vi "Wait on State.vi"(8 "error in (no error)":errorcluster, 9 "Timeout ms (-1)":i32=-1, 10 "Connection State":T1, 11 "VISA Client in":refnum<class "Serial Client.lvclass">) -> (0 "error out":errorcluster, 1 "Timed Out?":bool, 3 "VISA Client out":refnum<class "Serial Client.lvclass">)   [LabVIEW 2020, in "Stream-Serial.lvlib" / "Serial Client.lvclass"]
uses:
  Serial Client.lvclass
  Connection State.ctl
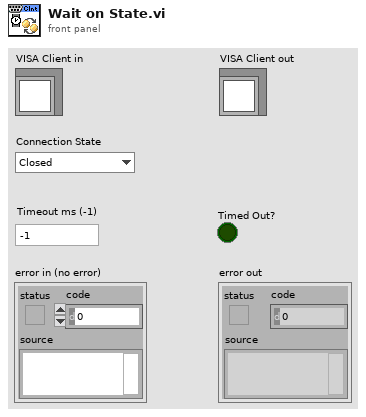
[diagram p1: front panel]
types:
  T1 = typedef "Stream-Serial.lvlib/Serial Client.lvclass/Connection State.ctl" = enum16{"Closed", "Idle", "Connecting", "Connected", "Shutdown"}
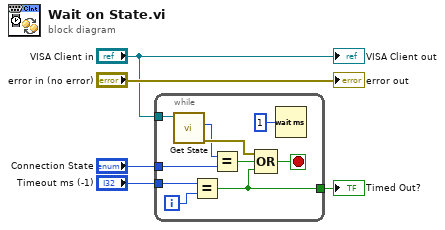
[diagram p0: block diagram]
diagram:
  n1 = while {
    tunnel: "VISA Client in" -> [w15]
    tunnel: "Connection State" -> [w10]
    tunnel: "Timeout ms (-1)" -> [w13]
    tunnel: [w6] -> w1
    i -> [w12]
    stop <- w7 stop-if-true
    n2 = call "Get State.vi"("VISA Client in"=w15) -> ("error out"=w11:errorcluster, "State"=w9:T1)  [unwired: 8 in, 1 out]
    n3 = Equal?(x=w13, y=w12) -> (x = y?=w6:bool)
    n4 = Equal?(x=w9, y=w10) -> (x = y?=w8:bool)
    n5 = Compound Arithmetic op=OR(w11, w8, w6) -> (w7:bool)
    n6 = Wait (ms)(milliseconds to wait=u32 1) -> ()  [unwired: 1 out]
  }
  "Timed Out?" <- w1
  "error out" <- "error in (no error)"
  "VISA Client out" <- "VISA Client in"
